vi "Begin.vi"(8 "error in":errorcluster) -> (0 "error out":errorcluster)   [LabVIEW 2017]
doc: "Called before other user functions, this VI can be used to open I/O refnums, load in file data, and do general program initialization. Notice that the <B>error out</B> terminal is simply used for data flow. Wiring it to other structures or subVIs ensures that this VI runs first."
uses:
  <vilib>/Rock Robotics/WPI/DriverStation/WPI_DriverStationRobotMode2.ctl
  <vilib>/Rock Robotics/WPI/Joystick/WPI_JoystickDeviceEnum.ctl
  <vilib>/Rock Robotics/WPI/ThirdParty/Phoenix-LabVIEW/Motor Controller/Controls/CTRE_Phoenix_MotorControl_FeedbackDevice.ctl
  <vilib>/Rock Robotics/SystemInterfaces/spilib/spi_bus.ctl
  <vilib>/Rock Robotics/WPI/Solenoid/WPI_SolenoidChannel.ctl
  <vilib>/Rock Robotics/WPI/Solenoid/WPI_SolenoidValue.ctl
  Odometry/Typedef/Odometry.ctl
  <vilib>/Rock Robotics/SystemInterfaces/DIO/FPGA_DIOChannel.ctl
  <vilib>/Rock Robotics/SystemInterfaces/DIO/FPGA_DIOPWMChannel.ctl
  Robot Global Data.vi
  <vilib>/Rock Robotics/Network Tables/NT Write String Array.vi
  <vilib>/Rock Robotics/WPI/Solenoid/WPI_SolenoidOpenDouble.vi
  <vilib>/Rock Robotics/WPI/Solenoid/WPI_SolenoidSetEnum.vi
  <vilib>/Rock Robotics/WPI/Counter/WPI_CounterDigitalInputToDigitalSource.vi
  <vilib>/Rock Robotics/WPI/MotorControl/WPI_MotorControlOpen TalonSRX.vi
  Drive/Implementation/Is High Gear.vi
  <vilib>/Rock Robotics/WPI/Counter/WPI_CounterEdgeLevel.ctl
  <vilib>/Rock Robotics/WPI/Accelerometer/WPI_AccelerometerRange.ctl
  <vilib>/Rock Robotics/WPI/Accelerometer/InternalAccelerometer/WPI_AccelerometerInternalOpen.vi
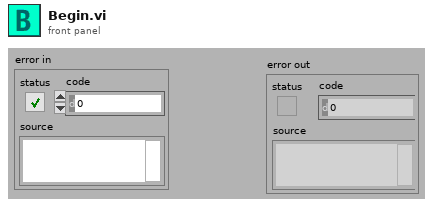
[diagram p1: front panel]
types:
  T1 = typedef "WPI_JoystickDeviceEnum.ctl" = enum16{"USB 0", "USB 1", "USB 2", "USB 3", "USB 4", "USB 5"}
  T2 = typedef "FPGA_DIOPWMChannel.ctl" = enum8{"PWM 0", "PWM 1", "PWM 2", "PWM 3", "PWM 4", "PWM 5", "PWM 6", "PWM 7", "PWM 8", "PWM 9", "PWM MXP 0", "PWM MXP 1", "PWM MXP 2", "PWM MXP 3", "PWM MXP 4", "PWM MXP 5", "PWM MXP 6", "PWM MXP 7", "PWM MXP 8", "PWM MXP 9", "Invalid"}
  T3 = typedef "FPGA_DIOChannel.ctl" = enum8{"DIO 0", "DIO 1", "DIO 2", "DIO 3", "DIO 4", "DIO 5", "DIO 6", "DIO 7", "DIO 8", "DIO 9", "DIO MXP 0", "DIO MXP 1", "DIO MXP 2", "DIO MXP 3", "DIO MXP 4", "DIO MXP 5", "DIO MXP 6", "DIO MXP 7", "DIO MXP 8", "DIO MXP 9", "DIO MXP 10", "DIO MXP 11", "DIO MXP 12", "DIO MXP 13", "DIO MXP 14", "DIO MXP 15", "SPI Port CS1", "SPI Port CS2", "SPI Port CS3", "SPI Port MISO", "SPI Port MOSI", "Invalid"}
  T4 = typedef "Odometry.ctl" = cluster{"x":dbl, "y":dbl, "theta":dbl, "Left Encoder Raw":i32, "Right Encoder Raw":i32, "Left Velocity Raw":i32, "Right Velocity Raw":i32, "Left Encoder":dbl, "Right Encoder":dbl, "Late Iterations":i16}
  T5 = cluster{"Kp":dbl, "Ki":dbl, "Kd":dbl, "Kf":dbl, "IZone":dbl}
  T6 = typedef "WPI_SolenoidValue.ctl" = enum16{"Off", "On", "Forward", "Reverse"}
  T7 = typedef "WPI_SolenoidChannel.ctl" = enum8{"Solenoid 0", "Solenoid 1", "Solenoid 2", "Solenoid 3", "Solenoid 4", "Solenoid 5", "Solenoid 6", "Solenoid 7", "Invalid"}
  T8 = typedef "spi_bus.ctl" = enum16{"SPI On-Board, CS0", "SPI On-Board, CS1", "SPI On-Board, CS2", "SPI On-Board, CS3", "SPI MXP", "Invalid"}
  T9 = typedef "CTRE_Phoenix_MotorControl_FeedbackDevice.ctl" = i8
  T10 = typedef "WPI_DriverStationRobotMode2.ctl" = enum16{"Autonomous Disabled", "Autonomous Enabled", "Teleop Disabled", "Teleop Enabled", "Disconnected", "Finish", "Test Disabled", "Test Enabled", "Emergency Stopped"}
  T11 = typedef "WPI_JoystickDevRef.ctl" = cluster{"Device":T1}
  T12 = typedef "WPI_AccelerometerRange.ctl" = enum16{"+/- 2 g", "+/- 4 g", "+/- 8 g"}
  T13 = typedef "WPI_AccelerometerDevRef.ctl" = cluster{"DevStatus":errorcluster, "Scaling":T14, "Analog Channels":T15, "I2C Bus":T17, "SPI Bus":T8, "Accel Range":T18, "ADXL Axes":T19, "Handle":i32, "Device Address":u8, "Accel Type":enum16{"Analog", "ADXL345 I2C", "ADXL345 SPI", "Internal", "ADXL362 SPI"}}
  T14 = typedef "WPI_AccelerometerScaling.ctl" = cluster{"Gain (VoltsPerG)":dbl, "Center Voltage":dbl}
  T15 = typedef "WPI_AccelerometerAnalogChannels.ctl" = cluster{"X-Axis":T16, "Y-Axis":T16, "Z-Axis":T16}
  T16 = typedef "FPGA_AIChannel.ctl" = enum8{"AI 0", "AI 1", "AI 2", "AI 3", "AI MXP 0", "AI MXP 1", "AI MXP 2", "AI MXP 3", "Invalid"}
  T17 = typedef "i2c_bus.ctl" = enum16{"I2C On-Board", "I2C MXP", "Invalid"}
  T18 = typedef "ADXL345 Range.ctl" = u8
  T19 = typedef "WPI_AccelerometerADXL345 Axes.ctl" = cluster{"X-Axis":bool, "Y-Axis":bool, "Z-Axis":bool}
  T20 = typedef "WPI_SolenoidDevRef.ctl" = cluster{"DevStatus":errorcluster, "Pneumatics Control Module":u8, "Forward Solenoid Channel":T7, "Reverse Solenoid Channel":T7}
  T21 = typedef "WPI_GyroDevRef.ctl" = cluster{"DevStatus":errorcluster, "Analog Channel":T16, "Gain (VoltsPerDegree/Second)":dbl, "Gyro Type":enum16{"Analog", "XRS450"}, "Handle":i32, "SPI Bus":T8, "Device Found":bool, "Sample Rate":dbl, "Calibrate On Open":bool, "Offset":dbl}
  T22 = typedef "TalonSRX6Motor.ctl" = cluster{"FrontLeftMaster":T23, "FrontLeftSlave1":T23, "FrontLeftSlave2":T23, "FrontRightMaster":T23, "FrontRightSlave1":T23, "FrontRightSlave2":T23}
  T23 = typedef "WPI_MotorControlDeviceRef.ctl" = cluster{"DeviceStatus":errorcluster, "Type":T24, "PWM":cluster{"PWM Channel":T2, "DeadBand":T25}, "CAN":cluster{"Device Number":u8, "SetOutput VI Ref":variant, "GetOutput VI Ref":variant, "Enable VI Ref":variant, "Disable VI Ref":variant, "Data":variant}, "Invert":bool, "DIO PWM":cluster{"PWM \"Enable\" Channel":T2, "DIOChannel":T3, "PWM Rate":dbl}}
  T24 = typedef "WPI_MotorControlType.ctl" = enum16{"PWM", "CAN", "DIO PWM"}
  T25 = typedef "WPI_PWMDeadband.ctl" = cluster{"Name":string, "maxPositivePwm":i32, "minPositivePwm":i32, "centerPwm":i32, "maxNegativePwm":i32, "minNegativePwm":i32, "angularRange":u16}
  T26 = typedef "WPI_DigitalInputDevRef.ctl" = cluster{"DevStatus":errorcluster, "DIO Channel":T3}
  T27 = typedef "WPI_CounterEdgeLevel.ctl" = enum16{"Active Low", "Active High", "Falling Edge", "Rising Edge"}
  T28 = typedef "FPGA_CounterEncoderSourceConvertionLVSourceType.ctl" = cluster{"DevStatus":errorcluster, "AnalogTriggerMode?":bool, "DigitalMode":cluster{"DIO Channel":T29}, "AnalogTriggerMode":cluster{"AnalogTriggerIndex":T30, "OutputType":T31}}
  T29 = typedef "FPGA_DIODigitalSourceChannel.ctl" = enum8{"DIO 0", "DIO 1", "DIO 2", "DIO 3", "DIO 4", "DIO 5", "DIO 6", "DIO 7", "DIO 8", "DIO 9", "DIO MXP 0", "DIO MXP 1", "DIO MXP 2", "DIO MXP 3", "DIO MXP 4", "DIO MXP 5", "DIO MXP 6", "DIO MXP 7", "DIO MXP 8", "DIO MXP 9", "DIO MXP 10", "DIO MXP 11", "DIO MXP 12", "DIO MXP 13", "DIO MXP 14", "DIO MXP 15", "Disabled"}
  T30 = typedef "FPGA_AnalogTriggerIndex.ctl" = enum8{"Trig 0", "Trig 1", "Trig 2", "Trig 3", "Trig 4", "Trig 5", "Trig 6", "Trig 7", "Invalid"}
  T31 = typedef "FPGA_AnalogTriggerOutType.ctl" = enum16{"InWindow", "TriggerState", "Rising", "Falling"}
  T32 = typedef "WPI_EncoderDevRef.ctl" = cluster{"DevStatus":errorcluster, "EncoderIndex":T33, "CounterIndex":T34, "DistancePerCount":dbl, "Decoding Type":T35}
  T33 = typedef "FPGA_EncoderIdx.ctl" = enum8{"Enc 0", "Enc 1", "Enc 2", "Enc 3", "Enc 4", "Enc 5", "Enc 6", "Enc 7", "Invalid"}
  T34 = typedef "FPGA_CounterCtrSystemIndex.ctl" = enum8{"Ctr 0", "Ctr 1", "Ctr 2", "Ctr 3", "Ctr 4", "Ctr 5", "Ctr 6", "Ctr 7", "Invalid"}
  T35 = typedef "WPI_EncoderType.ctl" = enum16{"1x", "2x", "4x"}
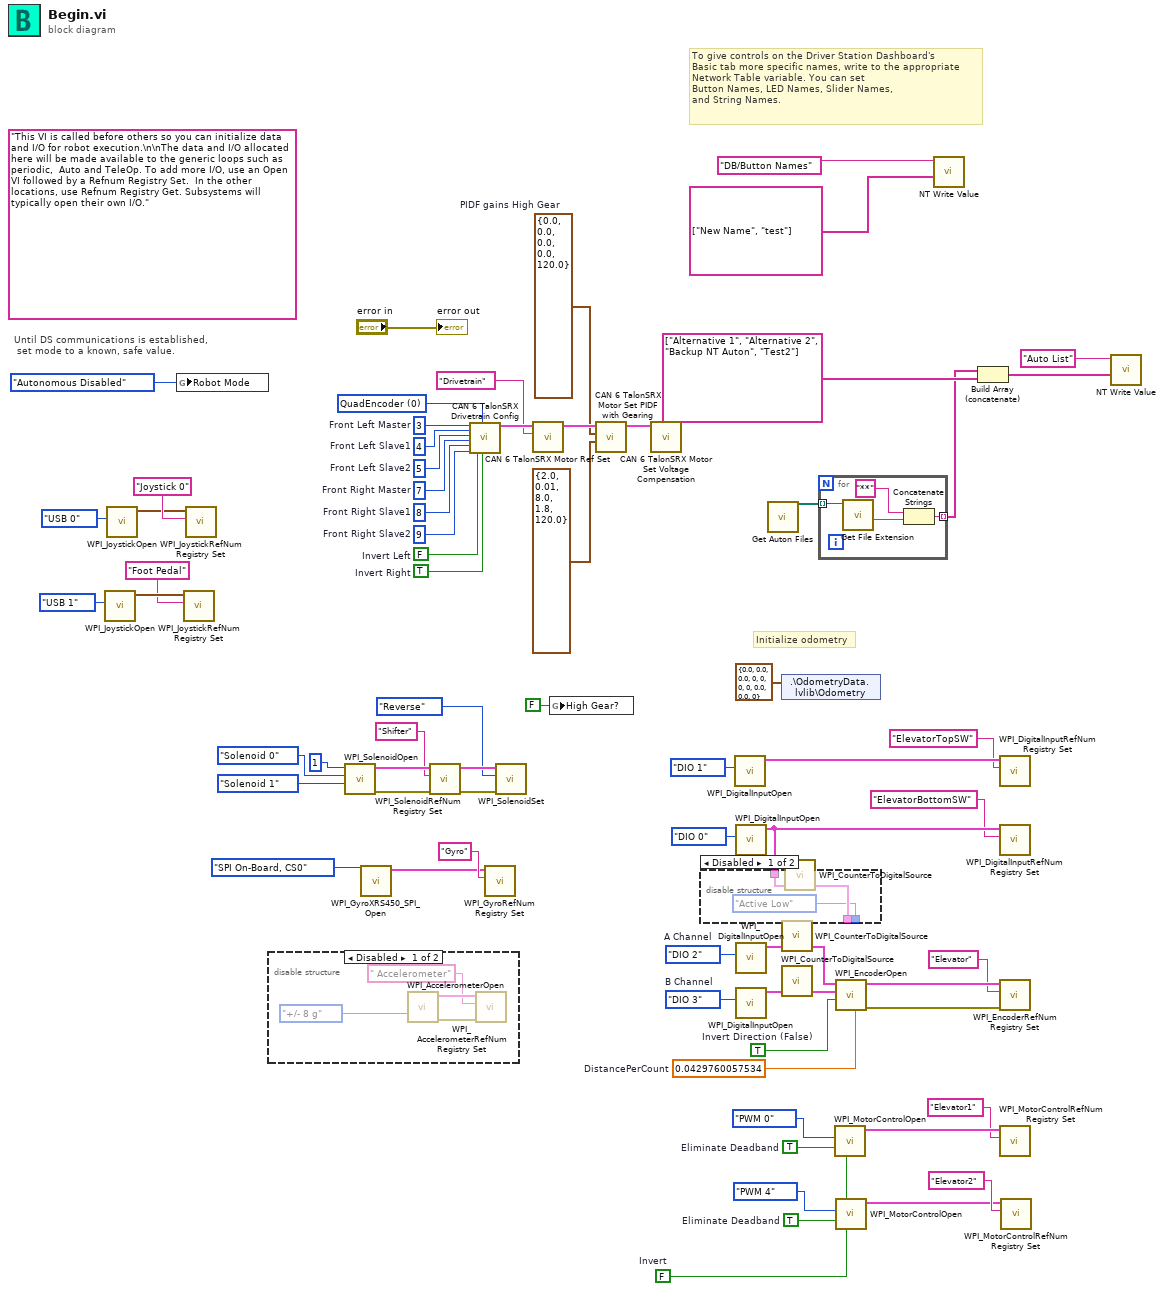
[diagram p0: block diagram]
diagram:
  w11 = FALSE  # Invert
  w15 = TRUE  # Eliminate Deadband
  w20 = TRUE  # Eliminate Deadband
  w28 = 0.0429760057534  # DistancePerCount
  w29 = TRUE  # Invert Direction (False)
  w38 = FPGA_DIOChannel."DIO 3"  # B Channel
  w37 = FPGA_DIOChannel."DIO 2"  # A Channel
  w40 = T5 {"Kp"=0.0, "Ki"=0.0, "Kd"=0.0, "Kf"=0.0, "IZone"=120.0}  # PIDF gains High Gear
  w54 = TRUE  # Invert Right
  w55 = T9 0 items=["None"=-1, "QuadEncoder"=0, "Analog"=2, "Tachometer"=4, "Pulse Width Encoded Position"=8, "Sensor Sum (S0 + S1)"=9, "Sensor Difference (D0 - D1)"=10, "Remote Source 0"=11, "Remote Source 1"=12, "Software Emulated"=15] ("Feedback Device")
  w56 = FALSE  # Invert Left
  w57 = u8 9  # Front Right Slave2
  w58 = u8 8  # Front Right Slave1
  w59 = u8 7  # Front Right Master
  w60 = u8 5  # Front Left Slave2
  w61 = u8 4  # Front Left Slave1
  w62 = u8 3  # Front Left Master
  (unwired) "This VI is called before others so you can initialize data and I/O for robot execution.\n\nThe data and I/O allocated here will be made available to the generic loops such as periodic,  Auto and TeleOp. To add more I/O, use an Open VI followed by a Refnum Registry Set.  In the other locations, use Refnum Registry Get. Subsystems will typically open their own I/O."
  # "Initialize odometry"
  # "To give controls on the Driver Station Dashboard's\nBasic tab more specific names, write to the appropriate\nNetwork Table variable. You can set\nButton Names, LED Names, Slider Names,\nand String Names."
  # "Until DS communications is established,\n set mode to a known, safe value."
  n1 = call <vilib>:"WPI_JoystickOpen.vi"("JoystickDevice"=WPI_JoystickDeviceEnum."USB 1") -> ("JoystickDevRef"=w9:T11)  [unwired: 10 in]
  n2 = call <vilib>:"WPI_JoystickOpen.vi"("JoystickDevice"=WPI_JoystickDeviceEnum."USB 0") -> ("JoystickDevRef"=w68:T11)  [unwired: 10 in]
  n3 = global write "Robot Global Data.vi" "Robot Mode"(WPI_DriverStationRobotMode2."Autonomous Disabled" ("Robot Mode")) -> ()
  n4 = call <vilib>:"WPI_JoystickRefNum Registry Set.vi"("refnum name"="Foot Pedal", "JoystickDevRef"=w9) -> ()  [unwired: 8 in, 2 out]
  n5 = call <vilib>:"WPI_JoystickRefNum Registry Set.vi"("refnum name"="Joystick 0", "JoystickDevRef"=w68) -> ()  [unwired: 8 in, 2 out]
  n6 = disable-structure shown="Disabled" {
    frame Disabled {
      n7 = call-poly <vilib>:"WPI_AccelerometerOpen.vi"("Accel Range"=WPI_AccelerometerRange."+/- 8 g") -> ("error out"=w72:errorcluster, "AccelerometerDevRef"=w73:T13)  [unwired: 9 in]
      n8 = call <vilib>:"WPI_AccelerometerRefNum Registry Set.vi"("error in (no error)"=w72, "refnum name"=" Accelerometer", "AccelerometerDevRef"=w73) -> ()  [unwired: 7 in, 2 out]
    }
    frame Enabled {
    }
  }
  n9 = call-poly <vilib>:"WPI_SolenoidOpen.vi"("Reverse Solenoid Channel"=WPI_SolenoidChannel."Solenoid 1", "Forward Solenoid Channel"=WPI_SolenoidChannel."Solenoid 0", "Pneumatics Control Module (0)"=u8 1) -> ("error out"=w47:errorcluster, "SolenoidDevRef"=w48:T20)  [unwired: 7 in]
  n10 = call <vilib>:"WPI_GyroXRS450_SPI_Open.vi"("SPI Bus"=spi_bus."SPI On-Board, CS0") -> ("GyroDevRef"=w12:T21)  [unwired: 8 in, 2 out]
  n11 = call <vilib>:"WPI_SolenoidRefNum Registry Set.vi"("error in (no error)"=w47, "refnum name"="Shifter", "SolenoidDevRef"=w48) -> ("error out"=w44:errorcluster, "SolenoidDevRef"=w45:T20)  [unwired: 7 in]
  n12 = call "CAN 6 TalonSRX Drivetrain Config.vi"("Front Left Master"=w62, "Front Left Slave1"=w61, "Front Left Slave2"=w60, "Front Right Master"=w59, "Front Right Slave1"=w58, "Front Right Slave2"=w57, "Invert Left"=w56, "Feedback Device"=w55, "Invert Right"=w54) -> ("TalonSRX6MotorRef"=w53:T22)  [unwired: 10 in]
  n13 = call <vilib>:"WPI_GyroRefNum Registry Set.vi"("refnum name"="Gyro", "GyroDevRef"=w12) -> ()  [unwired: 8 in, 2 out]
  n14 = call-poly <vilib>:"WPI_SolenoidSet.vi"("error in (no error)"=w44, "Value"=WPI_SolenoidValue."Reverse", "SolenoidDevRef"=w45) -> ()  [unwired: 7 in, 2 out]
  n15 = call "CAN 6 TalonSRX Motor Ref Set.vi"("refnum name"="Drivetrain", "TalonSRX6MotorRef in"=w53) -> ("TalonSRX6MotorRef out"=w42:T22)  [unwired: 8 in, 1 out]
  n16 = global write "Is High Gear.vi" "High Gear?"(FALSE ("High Gear?")) -> ()
  n17 = call "CAN 6 TalonSRX Motor Set PIDF with Gearing.vi"("PIDF gains Low Gear"=T5 {"Kp"=2.0, "Ki"=0.01, "Kd"=8.0, "Kf"=1.8, "IZone"=120.0}, "PIDF gains High Gear"=w40, "TalonSRX6MotorRef"=w42) -> ("TalonSRX6MotorRef"=w1:T22)  [unwired: 8 in]
  n18 = call "CAN 6 TalonSRX Motor Set Voltage Compensation.vi"("TalonSRX6MotorRef"=w1) -> ()  [unwired: 10 in, 1 out]
  n19 = call <vilib>:"WPI_DigitalInputOpen.vi"("DIO Channel"=FPGA_DIOChannel."DIO 1") -> ("DigitalInputDevRef"=w25:T26)  [unwired: 9 in, 1 out]
  n20 = call <vilib>:"WPI_DigitalInputOpen.vi"("DIO Channel"=FPGA_DIOChannel."DIO 0") -> ("DigitalInputDevRef"=w27:T26)  [unwired: 9 in, 1 out]
  n21 = disable-structure shown="Disabled" {
    disable-tunnel: [w77 _] -> _
    disable-tunnel: [WPI_CounterEdgeLevel."Active Low" ("External Reset Trigger") _] -> _
    disable-tunnel: w27 -> [w75 _]
    frame Disabled {
      n22 = call-poly <vilib>:"WPI_CounterToDigitalSource.vi"("DigitalInputDevRef"=w75) -> ("Digital Source"=w77:T28)  [unwired: 6 in]
    }
    frame Enabled {
    }
  }
  n23 = call <vilib>:"WPI_DigitalInputOpen.vi"("DIO Channel"=w37) -> ("DigitalInputDevRef"=w34:T26)  [unwired: 1 in, 9 out]
  n24 = call <vilib>:"WPI_DigitalInputOpen.vi"("DIO Channel"=w38) -> ("DigitalInputDevRef"=w35:T26)  [unwired: 1 in, 9 out]
  n25 = call "Get Auton Files.vi"() -> ("All Files in Dir"=w5:path[])  [unwired: 11 in]
  n26 = shared-variable ".\\OdometryData.lvlib\\Odometry"(T4 {"x"=0.0, "y"=0.0, "theta"=0.0, "Left Encoder Raw"=0, "Right Encoder Raw"=0, "Left Velocity Raw"=0, "Right Velocity Raw"=0, "Left Encoder"=0.0, "Right Encoder"=0.0, "Late Iterations"=0} ("Odometry")) -> ()  [unwired: 1 in, 1 out]
  n27 = call-poly <vilib>:"WPI_CounterToDigitalSource.vi"("DigitalInputDevRef"=w34) -> ("Digital Source"=w33:T28)  [unwired: 6 out]
  n28 = call-poly <vilib>:"WPI_CounterToDigitalSource.vi"("DigitalInputDevRef"=w35) -> ("Digital Source"=w36:T28)  [unwired: 6 out]
  n29 = for {
    tunnel: w5 -> [w81] mode=indexing
    tunnel: [w78] -> w4 mode=indexing
    n30 = call <vilib>:"Get File Extension.vi"("file"=w81) -> ("filename without extension"=w80:string)  [unwired: 6 in, 4 out]
    n31 = Concatenate Strings("**" ("string"), w80) -> (w78:string)
  }
  n32 = call-poly <vilib>:"WPI_MotorControlOpen.vi"("Invert"=w11, "Eliminate Deadband"=w20, "PWM Channel"=FPGA_DIOPWMChannel."PWM 0") -> ("MotorControlDeviceRef"=w19:T23)  [unwired: 7 in, 1 out]
  n33 = call <vilib>:"WPI_EncoderOpen.vi"("DistancePerCount"=w28, "Invert Direction (False)"=w29, "BSource"=w36, "ASource"=w33) -> ("error out"=w32:errorcluster, "EncoderDevRef"=w31:T32)  [unwired: 4 in, 2 out]
  n34 = call-poly <vilib>:"WPI_MotorControlOpen.vi"("Invert"=w11, "Eliminate Deadband"=w15, "PWM Channel"=FPGA_DIOPWMChannel."PWM 4") -> ("MotorControlDeviceRef"=w16:T23)  [unwired: 7 in, 1 out]
  n35 = call-poly <vilib>:"NT Write Value.vi"("String Array"=string[] ["New Name", "test"], "Name"="DB/Button Names") -> ()  [unwired: 9 in, 1 out]
  n36 = Build Array (concatenate)(w4, string[] ["Alternative 1", "Alternative 2", "Backup NT Auton", "Test2"] ("String Array")) -> (w3:string[])
  n37 = call <vilib>:"WPI_DigitalInputRefNum Registry Set.vi"("refnum name"="ElevatorTopSW", "DigitalInputDevRef"=w25) -> ()  [unwired: 8 in, 2 out]
  n38 = call <vilib>:"WPI_DigitalInputRefNum Registry Set.vi"("refnum name"="ElevatorBottomSW", "DigitalInputDevRef"=w27) -> ()  [unwired: 8 in, 2 out]
  n39 = call <vilib>:"WPI_EncoderRefNum Registry Set.vi"("error in (no error)"=w32, "refnum name"="Elevator", "EncoderDevRef"=w31) -> ()  [unwired: 7 in, 2 out]
  n40 = call <vilib>:"WPI_MotorControlRefNum Registry Set.vi"("refnum name"="Elevator1", "MotorControlDevRef"=w19) -> ()  [unwired: 8 in, 2 out]
  n41 = call <vilib>:"WPI_MotorControlRefNum Registry Set.vi"("refnum name"="Elevator2", "MotorControlDevRef"=w16) -> ()  [unwired: 8 in, 2 out]
  n42 = call-poly <vilib>:"NT Write Value.vi"("String Array"=w3, "Name"="Auto List") -> ()  [unwired: 9 in, 1 out]
  "error out" <- "error in"
